vi "lakeshore_336.vi"() -> ()   [LabVIEW 2020]
panel:
  in  "Command":string="*IDN?\n"
  out "read buffer":string
  in  "VISA resource name":refnum<visa-resource-name>
  # "LAKE SHORE 372"
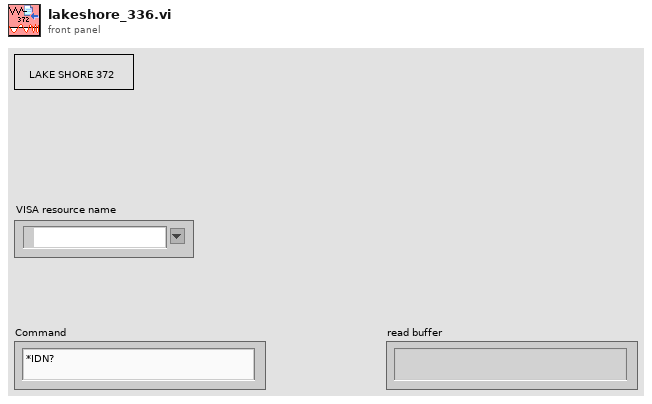
[diagram p1: front panel]
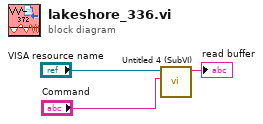
[diagram p0: block diagram]
diagram:
  n1 = call "Untitled 4 (SubVI).vi"("ID Query"="Command", "VISA Refnum in"="VISA resource name") -> ("read buffer"=→"read buffer":string)  [unwired: 9 in]
